vi "Overwrite-all-gui-parameters.vi"(8 "error in (no error)":errorcluster, 10 "Analys. params.":T1={"Binarization treshold"=120.0, "Image characteristics"=FALSE, "Melt-pool characteristics"=FALSE} {"Binarization treshold" min=0 max=255 step=1}, 11 "Analysis params. ref. in":refnum<data-value>) -> (0 "error out":errorcluster, 3 "Analysis params. ref.":refnum<data-value>)   [LabVIEW 2013, in "CameraVision.lvlib" / "CV-Analysis.lvclass"]
uses:
  CV-Analysis.lvclass
  Analysis-parameters-gui.ctl
  CV-Analysis.lvclass/CV-Analysis.ctl
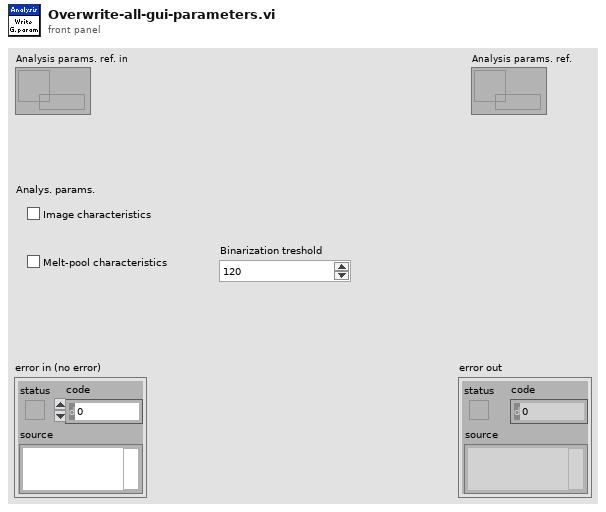
[diagram p1: front panel]
types:
  T1 = typedef "CameraVision.lvlib/CV-Analysis.lvclass/Analysis-parameters-gui.ctl" = cluster{"Binarization treshold":sgl, "Image characteristics":bool, "Melt-pool characteristics":bool}
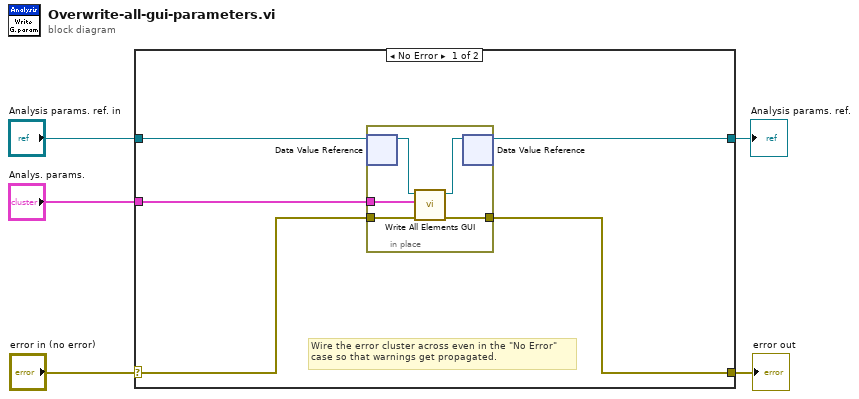
[diagram p0: block diagram]
diagram:
  n1 = case shown="No Error" "error in (no error)" {
    selector: "error in (no error)" -> [w9 w17]
    tunnel: [w8 w17] -> w4
    tunnel: "Analysis params. ref. in" -> [w7 w16]
    tunnel: "Analys. params." -> [w10 _]
    tunnel: [w6 w16] -> w1
    frame No Error {
      # "Wire the error cluster across even in the \"No Error\"\ncase so that warnings get propagated."
      n2 = in-place {
        in-place-border: w10 -> [w15]
        in-place-border: w9 -> [w14]
        in-place-border: [w13] -> w8
        n3 = in-place-dvr #1(w7) -> (w11:refnum<class "CV-Analysis.lvclass">)  [unwired: 1 out]
        n4 = call "Write All Elements GUI.vi"("error in (no error)"=w14, "Characteristics params."=w15, "Analysis params in"=w11) -> ("error out"=w13:errorcluster, "Analysis params out"=w12:refnum<class "CV-Analysis.lvclass">)  [unwired: 7 in]
        n5 = in-place-dvr #1(w12) -> (w6:refnum<data-value>)  [unwired: 1 out]
      }
    }
    frame Error {
    }
  }
  "error out" <- w4
  "Analysis params. ref." <- w1
